vi "ELVIS III v1.1 Open AI (N Samples).vi"(4 "Max Value":dbl[](array[numeric]), 6 "Min Value":dbl[](array[numeric]), 7 "Allow multiple opens?":bool, 8 "error in (no error)":errorcluster, 10 "Channel Names":string[](array[string]), 11 "Resource name":T7 caption="RIO Device") -> (0 "error out":errorcluster, 1 "AI (N Samples) Scale Constants List":T1, 2 "AI (N Samples) Channel List":T3, 3 "myRIO Ref Out":T5)   [LabVIEW 2021]
uses:
  <vilib>/userDefined/High Color/nirio_resource_hc.ctl
  <vilib>/myRIO/Common/Instrument Driver Framework/Utilities/typedefs/myRIO v1.0 Reference.ctl
  <vilib>/myRIO/Common/Instrument Driver Framework/Utilities/typedefs/Generic FPGA Reference.ctl
  <vilib>/myRIO/Common/Instrument Driver Framework/myRIO v1.0/AI Block/typedefs/AI Block Channels List.ctl
  <vilib>/myRIO/Common/Instrument Driver Framework/myRIO v1.0/AI Block/typedefs/AI Block Channels Enum.ctl
  <vilib>/myRIO/Common/Instrument Driver Framework/Utilities/typedefs/Analog Scaling Constants List.ctl
  <vilib>/myRIO/Common/Instrument Driver Framework/Utilities/typedefs/Analog Scaling Constants.ctl
  <vilib>/myRIO/Common/Instrument Driver Framework/ELVIS III v1.0/AI Block/typedefs/ELVIS III v1.0 AI Block Channels Enum.ctl
  <vilib>/Utility/VariantDataType/GetNumericInfo.vi
  <vilib>/Utility/error.llb/Error Cluster From Error Code.vi
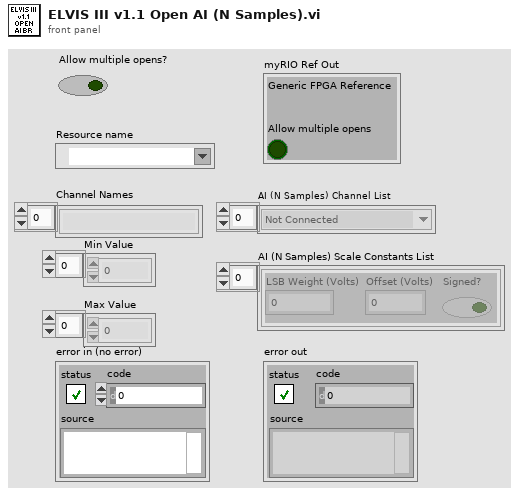
[diagram p1: front panel]
types:
  T1 = typedef "Analog Scaling Constants List.ctl" = T2[]
  T2 = typedef "Analog Scaling Constants.ctl" = cluster{"LSB Weight (Volts)":dbl, "Offset (Volts)":dbl, "Signed?":bool}
  T3 = typedef "AI Block Channels List.ctl" = T4[]
  T4 = typedef "AI Block Channels Enum.ctl" = enum16{"Not Connected", "A/AI0 (N Samples)", "A/AI1 (N Samples)", "A/AI2 (N Samples)", "A/AI3 (N Samples)", "A/AI4 (N Samples)", "A/AI5 (N Samples)", "A/AI6 (N Samples)", "A/AI7 (N Samples)", "A/AI0 (DIFF N Samples)", "A/AI1 (DIFF N Samples)", "A/AI2 (DIFF N Samples)", "A/AI3 (DIFF N Samples)", "B/AI0 (N Samples)", "B/AI1 (N Samples)", "B/AI2 (N Samples)", "B/AI3 (N Samples)", "B/AI4 (N Samples)", "B/AI5 (N Samples)", "B/AI6 (N Samples)", "B/AI7 (N Samples)", "B/AI0 (DIFF N Samples)", "B/AI1 (DIFF N Samples)", "B/AI2 (DIFF N Samples)", "B/AI3 (DIFF N Samples)"}
  T5 = typedef "myRIO v1.0 Reference.ctl" = cluster{"Generic FPGA Reference":T6, "Allow multiple opens":bool}
  T6 = typedef "Generic FPGA Reference.ctl" = refnum<k20>
  T7 = typedef "nirio_resource_hc.ctl" = tag
  T8 = typedef "ELVIS III v1.0 AI Block Channels Enum.ctl" = enum16{"Not Connected", "A/AI0 (N Samples)", "A/AI1 (N Samples)", "A/AI2 (N Samples)", "A/AI3 (N Samples)", "A/AI4 (N Samples)", "A/AI5 (N Samples)", "A/AI6 (N Samples)", "A/AI7 (N Samples)", "A/AI0 (DIFF N Samples)", "A/AI1 (DIFF N Samples)", "A/AI2 (DIFF N Samples)", "A/AI3 (DIFF N Samples)", "B/AI0 (N Samples)", "B/AI1 (N Samples)", "B/AI2 (N Samples)", "B/AI3 (N Samples)", "B/AI4 (N Samples)", "B/AI5 (N Samples)", "B/AI6 (N Samples)", "B/AI7 (N Samples)", "B/AI0 (DIFF N Samples)", "B/AI1 (DIFF N Samples)", "B/AI2 (DIFF N Samples)", "B/AI3 (DIFF N Samples)"}
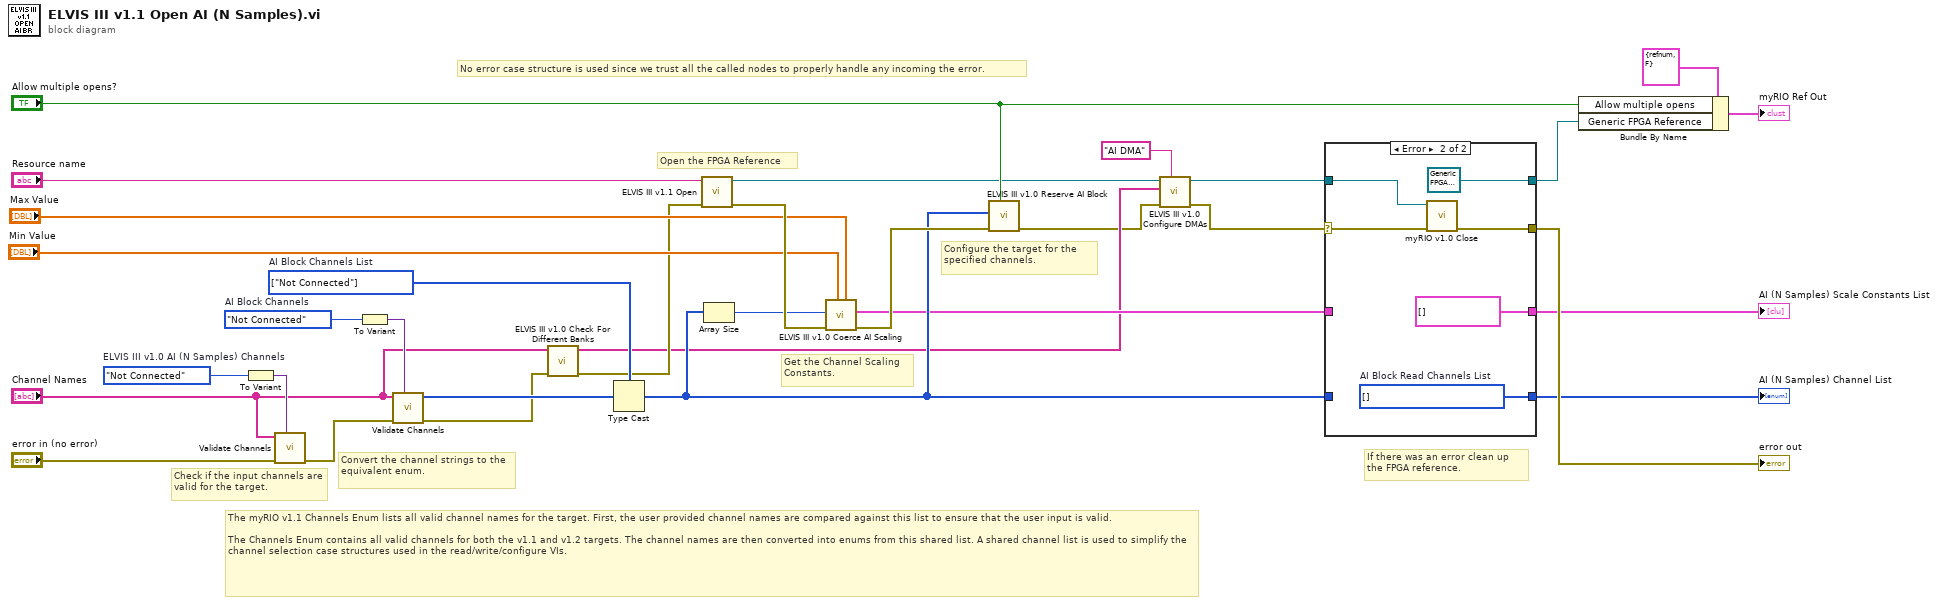
[diagram p0: block diagram]
diagram:
  w20 = T3 [enum."Not Connected"] items=["Not Connected", "A/AI0 (N Samples)", "A/AI1 (N Samples)", "A/AI2 (N Samples)", "A/AI3 (N Samples)", "A/AI4 (N Samples)", "A/AI5 (N Samples)", "A/AI6 (N Samples)", "A/AI7 (N Samples)", "A/AI0 (DIFF N Samples)", "A/AI1 (DIFF N Samples)", "A/AI2 (DIFF N Samples)", "A/AI3 (DIFF N Samples)", "B/AI0 (N Samples)", "B/AI1 (N Samples)", "B/AI2 (N Samples)", "B/AI3 (N Samples)", "B/AI4 (N Samples)", "B/AI5 (N Samples)", "B/AI6 (N Samples)", "B/AI7 (N Samples)", "B/AI0 (DIFF N Samples)", "B/AI1 (DIFF N Samples)", "B/AI2 (DIFF N Samples)", "B/AI3 (DIFF N Samples)"]  # AI Block Channels List
  w21 = AI_Block_Channels_Enum."Not Connected"  # AI Block Channels
  w22 = ELVIS_III_v1.0_AI_Block_Channels_Enum."Not Connected"  # ELVIS III v1.0 AI (N Samples) Channels
  # "Get the Channel Scaling Constants."
  # "The myRIO v1.1 Channels Enum lists all valid channel names for the target. First, the user provided channel names are compared against this list to ensure that the user input is valid.\n\nThe Channels Enum contains all valid channels for both the v1.1 and v1.2 targets. The channel names are then converted into enums from this shared list. A shared channel list is used to simplify the channel selection case structures used in the read/write/configure VIs."
  # "If there was an error clean up the FPGA reference."
  # "Configure the target for the specified channels."
  # "Open the FPGA Reference"
  # "No error case structure is used since we trust all the called nodes to properly handle any incoming the error."
  # "Convert the channel strings to the equivalent enum."
  # "Check if the input channels are valid for the target."
  n1 = To Variant(anything=w22) -> (Variant=w24:variant)
  n2 = call <vilib>:"Validate Channels.vi"("Channels Enum Variant"=w24, "error in (no error)"="error in (no error)", "Channel Names"="Channel Names") -> ("error out"=w30:errorcluster)  [unwired: 7 in, 1 out]
  n3 = To Variant(anything=w21) -> (Variant=w23:variant)
  n4 = call <vilib>:"Validate Channels.vi"("Channels Enum Variant"=w23, "error in (no error)"=w30, "Channel Names"="Channel Names") -> ("error out"=w8:errorcluster, "Index Array"=w27:u16[])  [unwired: 7 in]
  n5 = call <vilib>:"ELVIS III v1.0 Check For Different Banks.vi"("error in (no error)"=w8, "Channel Names"="Channel Names") -> ("error out"=w7:errorcluster)  [unwired: 9 in]
  n6 = Type Cast(type=w20, x=w27) -> (*(type *) &x=w13:T3)
  n7 = call <vilib>:"ELVIS III v1.1 Open.vi"("error in (no error)"=w7, "Resource name"="Resource name") -> ("error out"=w16:errorcluster, "myRIO FPGA Ref Out"=w3:T6)  [unwired: 8 in]
  n8 = Array Size(array=w13) -> (size(s)=w12:i32)
  n9 = call <vilib>:"ELVIS III v1.0 Coerce AI Scaling.vi"("Max Value"="Max Value", "Min Value"="Min Value", "error in (no error)"=w16, "Channel List Size"=w12) -> ("error out"=w15:errorcluster, "Scale Constants Array"=w11:T1)  [unwired: 6 in]
  n10 = call <vilib>:"ELVIS III v1.0 Reserve AI Block.vi"("Allow multiple opens?"="Allow multiple opens?", "error in (no error)"=w15, "AI (N Samples) Channels List"=w13) -> ("error out"=w5:errorcluster)  [unwired: 8 in]
  n11 = call <vilib>:"ELVIS III v1.0 Configure DMAs.vi"("DMA Type"="AI DMA", "error in (no error)"=w5, "Channel Names"="Channel Names", "ELVIS III FPGA Ref"=w3) -> ("error out"=w4:errorcluster, "ELVIS III FPGA Ref"=w2:T6)  [unwired: 6 in]
  n12 = case shown="Error" w4 {
    selector: w4 -> [w34 w41]
    tunnel: w2 -> [w35 w39]
    tunnel: [w35 T6 refnum ("myRIO FPGA Ref Out")] -> w25
    tunnel: [w34 w40] -> w28
    tunnel: [w33 w37] -> w19
    tunnel: w13 -> [w33 _]
    tunnel: w11 -> [w32 _]
    tunnel: [w32 T1 [] ("AI Block Read Scale Constants List")] -> w14
    frame No Error {
    }
    frame Error {
      w37 = T3 [] items=["Not Connected", "A/AI0 (N Samples)", "A/AI1 (N Samples)", "A/AI2 (N Samples)", "A/AI3 (N Samples)", "A/AI4 (N Samples)", "A/AI5 (N Samples)", "A/AI6 (N Samples)", "A/AI7 (N Samples)", "A/AI0 (DIFF N Samples)", "A/AI1 (DIFF N Samples)", "A/AI2 (DIFF N Samples)", "A/AI3 (DIFF N Samples)", "B/AI0 (N Samples)", "B/AI1 (N Samples)", "B/AI2 (N Samples)", "B/AI3 (N Samples)", "B/AI4 (N Samples)", "B/AI5 (N Samples)", "B/AI6 (N Samples)", "B/AI7 (N Samples)", "B/AI0 (DIFF N Samples)", "B/AI1 (DIFF N Samples)", "B/AI2 (DIFF N Samples)", "B/AI3 (DIFF N Samples)"]  # AI Block Read Channels List
      n13 = call <vilib>:"myRIO v1.0 Close.vi"("error in (no error)"=w41, "myRIO FPGA Ref In"=w39) -> ("error out"=w40:errorcluster)  [unwired: 9 in]
    }
  }
  "error out" <- w28
  "AI (N Samples) Channel List" <- w19
  "AI (N Samples) Scale Constants List" <- w14
  n14 = Bundle By Name(cluster=T5 {"Generic FPGA Reference"=refnum, "Allow multiple opens"=FALSE} ("myRIO Ref Out"), "Allow multiple opens"="Allow multiple opens?", "Generic FPGA Reference"=w25) -> (→"myRIO Ref Out":T5)
